vi "stepper_adc.vi"() -> ()   [LabVIEW 2015]
uses:
  !LabView/Control 4.ctl
  !LabView/Control 3.ctl
  !LabView/Control 2.ctl
  <vilib>/Instr/_visa.llb/VISA Configure Serial Port (Instr).vi
panel:
  out "Numeric":i32 format="%1d"
  out "Slide":u8(slide) scale=0.0..100.0
  out "ADC":dbl(graph)
  in  "Samples":T1=100
  in  "Steps in series":T2=100
  in  "file (use dialog)":path=path "C:/adc.txt"
  in  "Number of plots":T3=100
  out "ADC data":string
  in  "ADC port":refnum<visa-resource-name>="COM7"
  in  "Stepper port":refnum<visa-resource-name>="COM9"
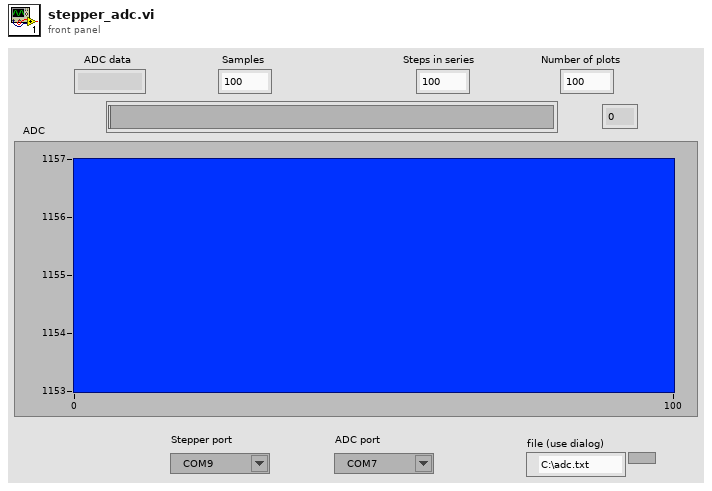
[diagram p1: front panel]
types:
  T1 = typedef "Control 2.ctl" = u16
  T2 = typedef "Control 3.ctl" = u32
  T3 = typedef "Control 4.ctl" = u32
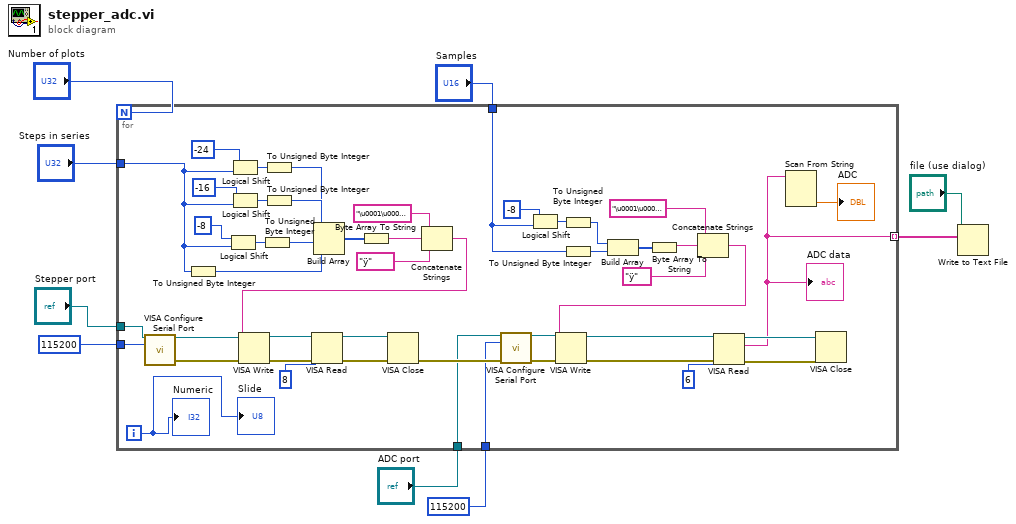
[diagram p0: block diagram]
diagram:
  n1 = for {
    N: "Number of plots" -> [_]
    tunnel: [w45] -> w8 mode=indexing
    tunnel: "Steps in series" -> [w19]
    tunnel: "Stepper port" -> [w18]
    tunnel: u32 115200 ("baud rate (115200)") -> [w17]
    tunnel: "Samples" -> [w15]
    tunnel: "ADC port" -> [w14]
    tunnel: u32 115200 ("baud rate (115200)") -> [w13]
    i -> [w10]
    n2 = call-poly "VISA Configure Serial Port"("VISA resource name"=w18, "baud rate (9600)"=w17) -> ("VISA resource name out"=w22:refnum<visa-resource-name>, "error out"=w21:errorcluster)  [unwired: 12 in]
    n3 = To Unsigned Byte Integer(number=w19) -> (unsigned 8bit integer=w42:u8)
    n4 = Logical Shift(y=i16 -8, x=w19) -> (x << y=w43:T2)
    n5 = Logical Shift(y=i16 -24, x=w19) -> (x << y=w32:T2)
    n6 = Logical Shift(y=i16 -16, x=w19) -> (x << y=w34:T2)
    n7 = To Unsigned Byte Integer(number=w43) -> (unsigned 8bit integer=w40:u8)
    n8 = To Unsigned Byte Integer(number=w32) -> (unsigned 8bit integer=w31:u8)
    n9 = To Unsigned Byte Integer(number=w34) -> (unsigned 8bit integer=w33:u8)
    n10 = Build Array(w31, w33, w40, w42) -> (w41:u8[])
    n11 = Byte Array To String(unsigned byte array=w41) -> (string=w35:string)
    n12 = Concatenate Strings("\u0001\u0000\u0000" ("string"), w35, "ÿ" ("string")) -> (w20:string)
    n13 = VISA Write(VISA resource name=w22, write buffer=w20, error in (no error)=w21) -> (VISA resource name out=w57:refnum<visa-resource-name>, error out=w56:errorcluster)  [unwired: 1 out]
    n14 = VISA Read(VISA resource name=w57, byte count=u32 8, error in (no error)=w56) -> (VISA resource name out=w50:refnum<visa-resource-name>, error out=w49:errorcluster)  [unwired: 2 out]
    n15 = VISA Close(VISA resource name=w50, error in (no error)=w49) -> (error out=w46:errorcluster)
    n16 = call-poly "VISA Configure Serial Port"("VISA resource name"=w14, "baud rate (9600)"=w13, "error in (no error)"=w46) -> ("VISA resource name out"=w48:refnum<visa-resource-name>, "error out"=w47:errorcluster)  [unwired: 11 in]
    n17 = Logical Shift(y=i16 -8, x=w15) -> (x << y=w30:T1)
    n18 = To Unsigned Byte Integer(number=w30) -> (unsigned 8bit integer=w28:u8)
    n19 = To Unsigned Byte Integer(number=w15) -> (unsigned 8bit integer=w27:u8)
    n20 = Build Array(w28, w27) -> (w26:u8[])
    n21 = Byte Array To String(unsigned byte array=w26) -> (string=w25:string)
    n22 = Concatenate Strings("\u0001\u0000\u0000" ("string"), w25, "ÿ" ("string")) -> (w12:string)
    n23 = VISA Write(VISA resource name=w48, write buffer=w12, error in (no error)=w47) -> (VISA resource name out=w55:refnum<visa-resource-name>, error out=w54:errorcluster)  [unwired: 1 out]
    n24 = VISA Read(VISA resource name=w55, byte count=u32 6, error in (no error)=w54) -> (VISA resource name out=w52:refnum<visa-resource-name>, read buffer=w45:string, error out=w51:errorcluster)  [unwired: 1 out]
    "ADC data" <- w45
    n25 = Scan From String(input string=w45) -> (output 1=→"ADC":dbl)  [unwired: 4 in, 3 out]
    n26 = VISA Close(VISA resource name=w52, error in (no error)=w51) -> ()  [unwired: 1 out]
    "Slide" <- w10
    "Numeric" <- w10
  }
  n27 = Write to Text File(file (use dialog)="file (use dialog)", text=w8) -> ()  [unwired: 2 in, 3 out]
